vi "GetParam.vi"(8 "error in (no error)":errorcluster caption="entrée d'erreur (pas d'erreur)", 11 "Contingency_Matrix.lvclass":refnum<class "Contingency_Matrix.lvclass">) -> (0 "error out":errorcluster caption="sortie d'erreur", 2 "contingency_matrix":cluster{"eps":string, "sparse":bool}={"eps"="None", "sparse"=FALSE}, 3 "Contingency_Matrix.lvclass":refnum<class "Contingency_Matrix.lvclass">)   [LabVIEW 2020, in "Contingency_Matrix.lvclass"]
doc: "Get Parameters"
uses:
  Contingency_Matrix.lvclass
  Contingency_Matrix.lvclass/Contingency_Matrix.ctl
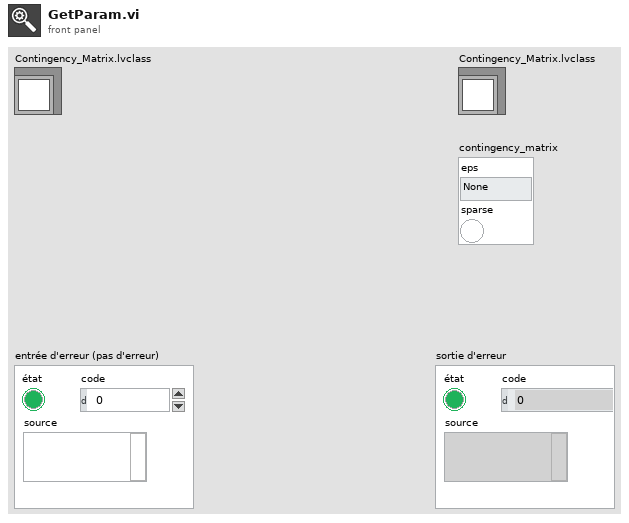
[diagram p1: front panel]
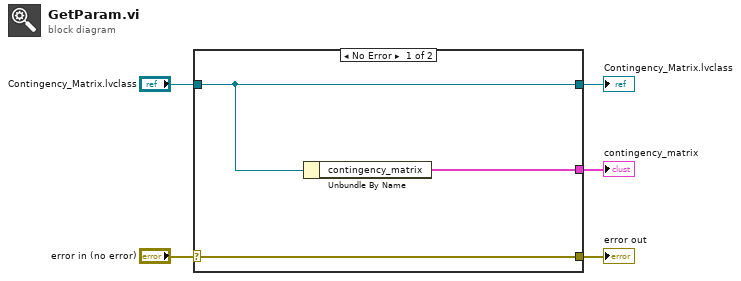
[diagram p0: block diagram]
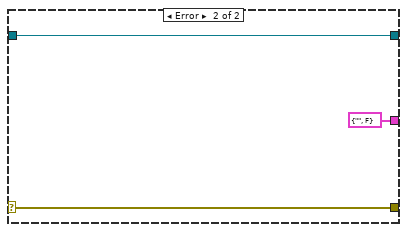
[diagram p2: hidden frame]
diagram:
  n1 = case shown="No Error" "error in (no error)" {
    selector: "error in (no error)" -> [w8 w10]
    tunnel: [w8 w10] -> w4
    tunnel: [w7 w11] -> w2
    tunnel: "Contingency_Matrix.lvclass" -> [w7 w11]
    tunnel: [w6 cluster{"eps":string, "sparse":bool} {"eps"="", "sparse"=FALSE} ("contingency_matrix")] -> w1
    frame No Error {
      n2 = Unbundle By Name(w7) -> ("contingency_matrix"=w6:cluster{"eps":string, "sparse":bool})
    }
    frame Error {
    }
  }
  "error out" <- w4
  "Contingency_Matrix.lvclass" <- w2
  "contingency_matrix" <- w1
